vi "IV_Sweep_multiple_stage.vi"() -> ()   [LabVIEW 2016]
uses:
  <instrlib>/Keithley 24XX/Public/Data/Read (Single Point).vi
  <instrlib>/Keithley 24XX/Keithley 24XX.lvlib
  <vilib>/Analysis/NI_AALPro.lvlib
panel:
  out "intercept":dbl
  out "slope":dbl
  in  "Source Mode  (0: Voltage)":u16(ring) items=["Voltage", "Current"]
  out "Steps (mV/uA)":dbl[](array[numeric])
  in  "Compliance  Level (A/V)":dbl=0.1
  out "IR":cluster{dbl[], dbl[]}(graph)
  out "VR":cluster{dbl[], dbl[]}(graph)
  in  "Delay Time (s)":dbl=1.0
  out "Resistance":sgl=-680628800000.0
  out "Current":sgl=-1.469503e-10
  out "Voltage":sgl=100.0186
  out "IV":cluster{dbl[], dbl[]}(graph)
  in  "Output filename":path
  in  "Start(V/mA)":dbl
  in  "End (mV/uA)":dbl[](array[numeric])
  in  "Interval (mV/uA)":dbl[](array[numeric])
  in  "2wire(F)/4wire(T)":bool
  in  "Enable Resistance Auto Range (T:Enable)":bool=TRUE
  in  "Enable Current Auto Range (T:Enable)":bool=TRUE
  in  "Enable Voltage Auto Range (T:Enable)":bool=TRUE
  in  "Resistance Manual Range (1.0)":dbl=1.0
  in  "Current Manual Range (1.0)":dbl=1.0
  in  "Voltage Manual Range (1.0)":dbl=1.0
  in  "Serial Configuration":T1={"Baud Rate"=9600, "Parity"=0, "Data Bits"=8, "Stop Bits"=10, "Flow Control"=0} {"Flow Control" items=["None", "XON/XOFF", "RTS/CTS", "XON/XOFF & RTS/CTS", "DTR/DSR", "XON/XOFF & DTR/DSR"]; "Stop Bits" items=["1.0"=10, "1.5"=15, "2.0"=20]; "Data Bits" items=["7"=7, "8"=8]; "Parity" items=["None", "Odd", "Even", "Mark", "Space"]; "Baud Rate" items=["300"=300, "600"=600, "1200"=1200, "2400"=2400, "4800"=4800, "9600"=9600, "19200"=19200]}
  in  "VISA resource name":refnum<visa-resource-name>="COM5"
  # "V-I"
  # "R-V"
  # "R-I"
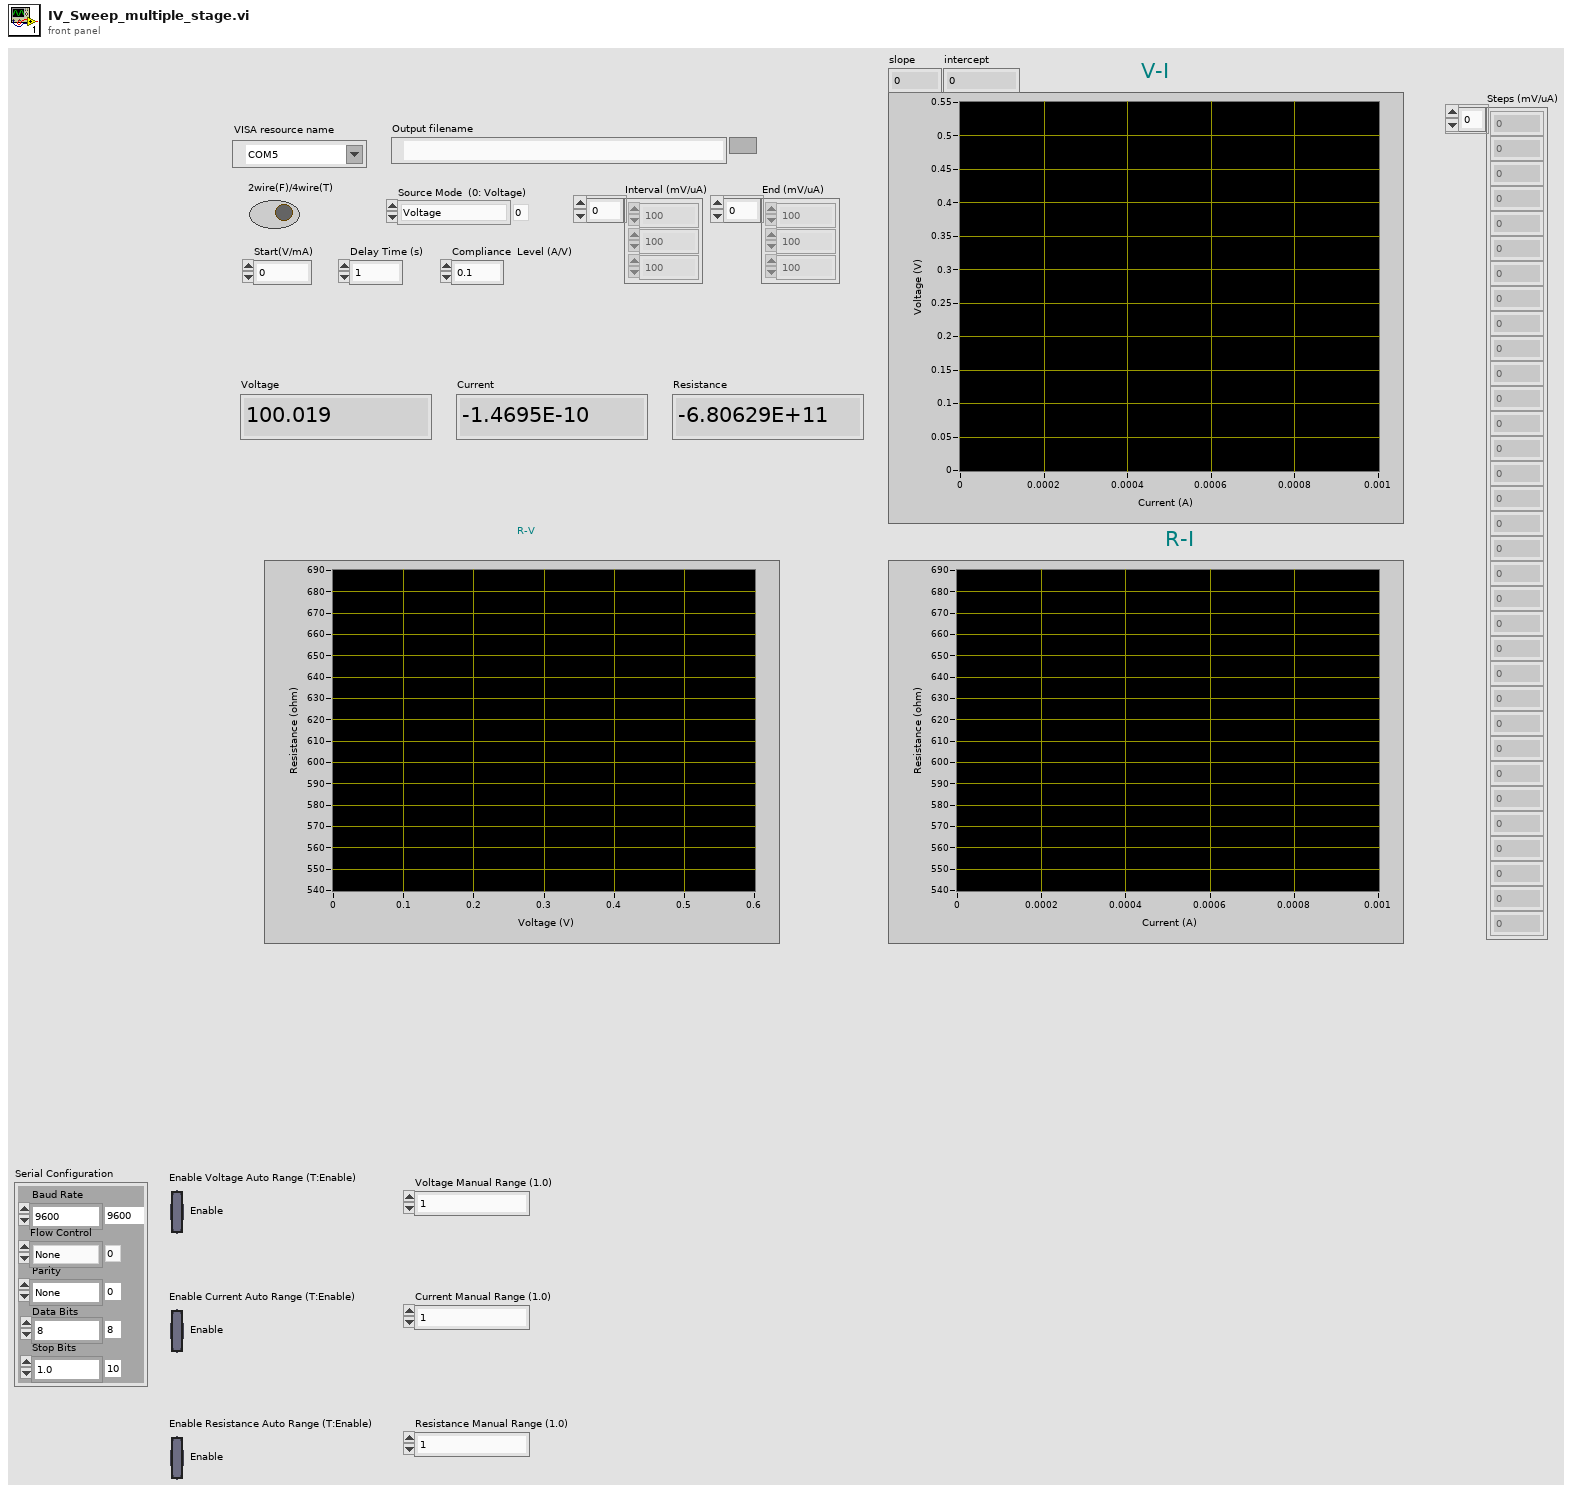
[diagram p1: front panel]
types:
  T1 = cluster{"Baud Rate":u32, "Parity":u16, "Data Bits":u16, "Stop Bits":u16, "Flow Control":u16}
  T2 = enum16{"open", "replace", "create", "open or create", "replace or create", "replace or create with confirmation"}
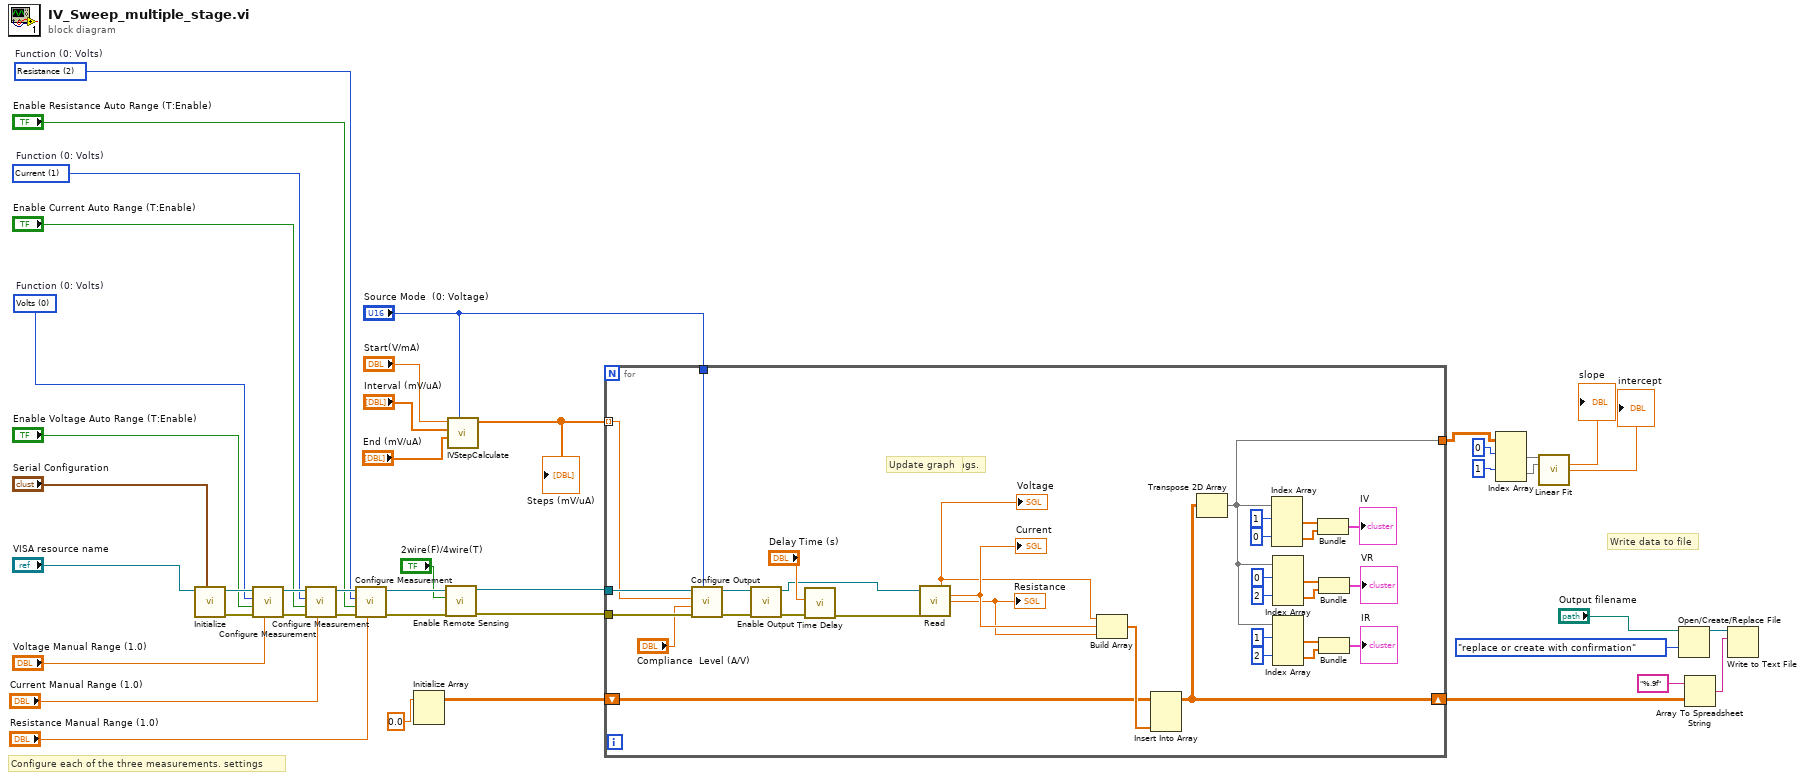
[diagram p0: block diagram]
diagram:
  w32 = u16 2 items=["Volts", "Current", "Resistance"]  # Function (0: Volts)
  w33 = u16 1 items=["Volts", "Current", "Resistance"]  # Function (0: Volts)
  w34 = u16 0 items=["Volts", "Current", "Resistance"]  # Function (0: Volts)
  # "Write data to file"
  # "Configure each of the three measurements. settings"
  n1 = call <instrlib>:"Initialize.vi"("Serial Configuration"="Serial Configuration", "VISA resource name"="VISA resource name") -> ("error out"=w39:errorcluster, "VISA resource name out"=w40:refnum<visa-resource-name>)  [unwired: 8 in]
  n2 = call <instrlib>:"Configure Measurement.vi"("Manual Range (1.0)"="Voltage Manual Range (1.0)", "error in (no error)"=w39, "Enable Auto Range (T:Enable)"="Enable Voltage Auto Range (T:Enable)", "Function (0: Volts)"=w34, "VISA resource name"=w40) -> ("error out"=w37:errorcluster, "VISA resource name out"=w38:refnum<visa-resource-name>)  [unwired: 5 in]
  n3 = call <instrlib>:"Configure Measurement.vi"("Manual Range (1.0)"="Current Manual Range (1.0)", "error in (no error)"=w37, "Enable Auto Range (T:Enable)"="Enable Current Auto Range (T:Enable)", "Function (0: Volts)"=w33, "VISA resource name"=w38) -> ("error out"=w36:errorcluster, "VISA resource name out"=w35:refnum<visa-resource-name>)  [unwired: 5 in]
  n4 = call <instrlib>:"Configure Measurement.vi"("Manual Range (1.0)"="Resistance Manual Range (1.0)", "error in (no error)"=w36, "Enable Auto Range (T:Enable)"="Enable Resistance Auto Range (T:Enable)", "Function (0: Volts)"=w32, "VISA resource name"=w35) -> ("error out"=w22:errorcluster, "VISA resource name out"=w23:refnum<visa-resource-name>)  [unwired: 5 in]
  n5 = Initialize Array(0.0 ("element")) -> (w24:dbl[][])  [unwired: 2 in]
  n6 = call <instrlib>:"Enable Remote Sensing.vi"("error in (no error)"=w22, "Enable Remote Sensing (T: Enable)"="2wire(F)/4wire(T)", "VISA resource name"=w23) -> ("error out"=w20:errorcluster, "VISA resource name out"=w21:refnum<visa-resource-name>)  [unwired: 7 in]
  n7 = call "IVStepCalculate.vi"("V(0)/I(1)"="Source Mode  (0: Voltage)", "End"="End (mV/uA)", "Interval"="Interval (mV/uA)", "Start"="Start(V/mA)") -> ("mV/uA"=w15:dbl[])  [unwired: 7 in]
  "Steps (mV/uA)" <- w15
  n8 = for {
    tunnel: w20 -> [w74]
    tunnel: w21 -> [w75]
    shift-right: [w46] -> w9
    shift-left: w24 -> [w50]
    tunnel: w15 -> [w45] mode=indexing
    tunnel: "Source Mode  (0: Voltage)" -> [w44]
    tunnel: [w43] -> w7
    # "Update graph"
    # "Take the readings."
    n9 = call <instrlib>:"Configure Output.vi"("Source Mode  (0: Voltage)"=w44, "error in (no error)"=w74, "Compliance  Level (0.1)"="Compliance  Level (A/V)", "Output Level (0)"=w45, "VISA resource name"=w75) -> ("error out"=w49:errorcluster, "VISA resource name out"=w48:refnum<visa-resource-name>)  [unwired: 5 in]
    n10 = call <instrlib>:"Enable Output.vi"("error in (no error)"=w49, "VISA resource name"=w48) -> ("error out"=w63:errorcluster, "VISA resource name out"=w64:refnum<visa-resource-name>)  [unwired: 8 in]
    n11 = call "Time Delay"("error in (no error)"=w63, "Delay Time (s)"="Delay Time (s)") -> ("error out"=w67:errorcluster)  [unwired: 9 in]
    n12 = call-poly <instrlib>:"Read.vi"("VISA resource name"=w64, "error in (no error)"=w67) -> ("Voltage"=w68:sgl, "Current"=w69:sgl, "Resistance"=w65:sgl)  [unwired: 7 in, 4 out]
    "Voltage" <- w68
    "Current" <- w69
    "Resistance" <- w65
    n13 = Build Array(w68, w69, w65) -> (w70:sgl[])
    n14 = Insert Into Array(array=w50, new element=w70) -> (w46:dbl[][])  [unwired: 2 in]
    n15 = Transpose 2D Array(2D array=w46) -> (transposed array=w43:dbl[][])
    n16 = Index Array(array=w43, index (row) #1=1 ("index (row)"), index (row) #2=0 ("index (row)")) -> (element #1=w72:dbl[], element #2=w73:dbl[])  [unwired: 2 in]
    n17 = Index Array(array=w43, index (row) #1=0 ("index (row)"), index (row) #2=2 ("index (row)")) -> (element #1=w59:dbl[], element #2=w60:dbl[])  [unwired: 2 in]
    n18 = Index Array(array=w43, index (row) #1=1 ("index (row)"), index (row) #2=2 ("index (row)")) -> (element #1=w54:dbl[], element #2=w55:dbl[])  [unwired: 2 in]
    n19 = Bundle(w72, w73) -> (→"IV":cluster{dbl[], dbl[]})  [unwired: 1 in]
    n20 = Bundle(w59, w60) -> (→"VR":cluster{dbl[], dbl[]})  [unwired: 1 in]
    n21 = Bundle(w54, w55) -> (→"IR":cluster{dbl[], dbl[]})  [unwired: 1 in]
  }
  n22 = Index Array(array=w7, index (row) #1=0 ("index (page)"), index (row) #2=1 ("index (row)")) -> (element #1=w4:dbl[], element #2=w3:dbl[])  [unwired: 2 in]
  n23 = call <vilib>:"Linear Fit.vi"("Y"=w4, "X"=w3) -> ("slope"=→"slope":dbl, "intercept"=→"intercept":dbl)  [unwired: 9 in, 3 out]
  n24 = Open/Create/Replace File(file path (use dialog)="Output filename", operation (0:open)=T2."replace or create with confirmation") -> (refnum out=w13:refnum<file>)  [unwired: 4 in, 2 out]
  n25 = Array To Spreadsheet String(array=w9, 3:"%.9f" ("format string")) -> (spreadsheet string=w10:string)  [unwired: 1 in]
  n26 = Write to Text File(file (use dialog)=w13, text=w10) -> ()  [unwired: 2 in, 3 out]
